vi "Check_for_Parent_Apply.vi"(8 "error in (no error)":errorcluster, 10 "AB_Source in":refnum<class "AB_Source.lvclass">, 11 "sourceItems in":refnum<class "AB_Source.lvclass">[](array[class])) -> (0 "error out":errorcluster, 1 "applyDestination":bool, 2 "applyInclusion":bool, 3 "sourceItems out":refnum<class "AB_Source.lvclass">[](array[class]), 4 "applyPassword":bool, 5 "applyProperties":bool)   [LabVIEW 2020, in "AB_Source.lvclass"]
uses:
  <vilib>/AppBuilder/AB_Classes/Source/AB_Source.lvclass
  <vilib>/AppBuilder/AB_Classes/Source/AB_Source.lvclass/AB_Source.ctl
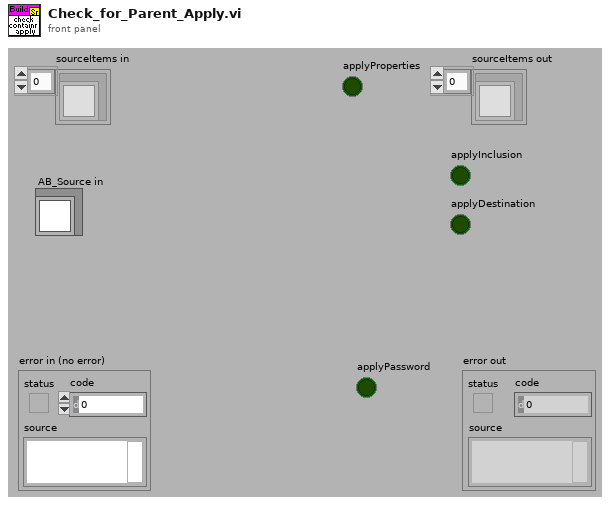
[diagram p1: front panel]
types:
  T1 = typedef "AB_Parent_Applies.ctl" = cluster{"inclusion":bool, "destination":bool, "properties":bool, "password":bool, "prefix":bool, "saveSettings":bool}
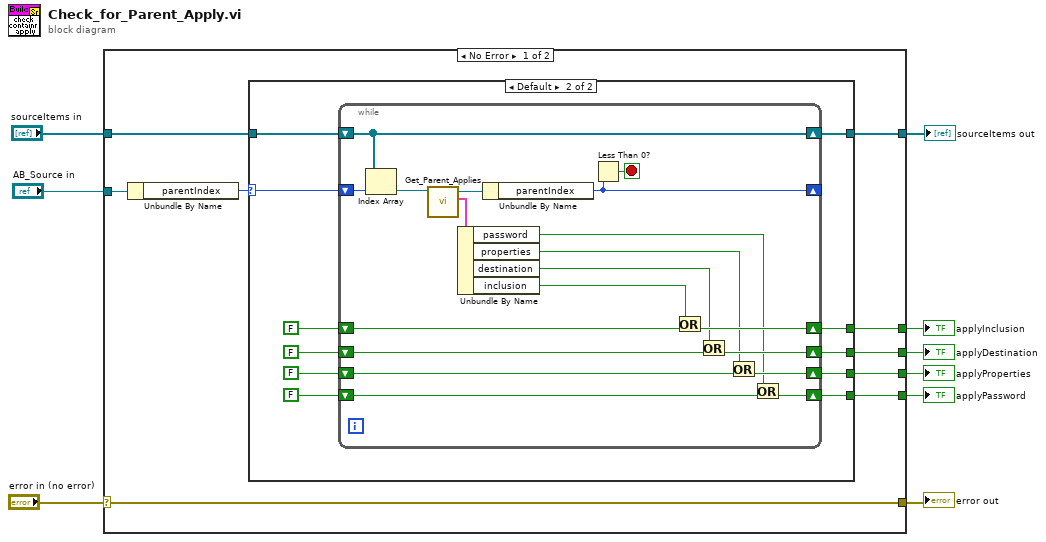
[diagram p0: block diagram]
diagram:
  n1 = case shown="No Error" "error in (no error)" {
    selector: "error in (no error)" -> [w18 w51]
    tunnel: [w18 w51] -> w8
    tunnel: "AB_Source in" -> [w11 _]
    tunnel: "sourceItems in" -> [w17 w50]
    tunnel: [w16 w50] -> w5
    tunnel: [w15 _] -> w4
    tunnel: [w14 _] -> w3
    tunnel: [w13 _] -> w2
    tunnel: [w12 _] -> w1
    frame No Error {
      n2 = Unbundle By Name(w11) -> ("parentIndex"=w10:i32)
      n3 = case shown="Default" w10 {
        selector: w10 -> [_ w30]
        tunnel: w17 -> [w19 w29]
        tunnel: [w19 w28] -> w16
        tunnel: [_ w23] -> w15
        tunnel: [_ w22] -> w14
        tunnel: [_ w21] -> w13
        tunnel: [_ w20] -> w12
        frame -1 {
        }
        frame Default {
          n4 = while {
            shift-right: [w38] -> _
            shift-left: w30 -> [w49]
            shift-right: [w45] -> w23
            shift-left: FALSE -> [w46]
            shift-right: [w47] -> w28
            shift-left: w29 -> [w47]
            shift-right: [w44] -> w22
            shift-left: FALSE -> [w43]
            shift-right: [w41] -> w21
            shift-left: FALSE -> [w42]
            shift-right: [w40] -> w20
            shift-left: FALSE -> [w39]
            stop <- w48 stop-if-true
            n5 = Index Array(array=w47, index=w49) -> (element=w33:refnum<class "AB_Source.lvclass">)
            n6 = call-dynamic "Get_Parent_Applies.vi"("AB_Source in"=w33) -> ("parentApplies"=w31:T1, "AB_Source out"=w32:refnum<class "AB_Source.lvclass">)  [unwired: 8 in, 1 out]
            n7 = Unbundle By Name(w31) -> ("password"=w37:bool, "properties"=w36:bool, "destination"=w35:bool, "inclusion"=w34:bool)
            n8 = Unbundle By Name(w32) -> ("parentIndex"=w38:i32)
            n9 = Less Than 0?(x=w38) -> (x < 0?=w48:bool)
            n10 = Or(x=w34, y=w46) -> (x .or. y?=w45:bool)
            n11 = Or(x=w35, y=w43) -> (x .or. y?=w44:bool)
            n12 = Or(x=w36, y=w42) -> (x .or. y?=w41:bool)
            n13 = Or(x=w37, y=w39) -> (x .or. y?=w40:bool)
          }
        }
      }
    }
    frame Error {
    }
  }
  "error out" <- w8
  "sourceItems out" <- w5
  "applyProperties" <- w2
  "applyPassword" <- w1
  "applyDestination" <- w3
  "applyInclusion" <- w4
